vi "EditOptions.vi"(8 "error in":errorcluster, 11 "SequenceNode in":refnum<class "CleanupCategoryNode.lvclass">) -> (0 "error out":errorcluster, 1 "edit options":T1, 2 "subnodes class":T2, 3 "SequenceNode out":refnum<class "CleanupCategoryNode.lvclass">)   [LabVIEW 2015, in "CleanupCategoryNode.lvclass"]
doc: "This VI Contains the options for the Menu that will be displayed when doing right click on an item\nThe subnodes class configures which nodes can be added to this nodes\nAnd the edit options determine which options are available for the node.\n\nThis configuration is stored in this VI in case some dynamic configuration is required for the menu options or subnodes.\n\nAll VIs must overide this methodCopyright 2017 National Instruments Corporation\n\nLicensed under the Apache License, Version 2.0 (the \"License\"); you may not use this file except in compliance with the License. You may obtain a copy of the License at http://www.apache.org/licenses/LICENSE-2.0\nUnless required by applicable law or agreed to in writing, software distributed under the License is distributed on an \"AS IS\" BASIS, WITHOUT WARRANTIES OR CONDITIONS OF ANY KIND, either express or implied. See the License for the specific language governing permissions and limitations under the License."
uses:
  CleanupCategoryNode.lvclass
  <vilib>/NI/Configuration Framework/Node/SubNodeCluster.ctl
  <vilib>/NI/Configuration Framework/Node/NodeMenuOptions.ctl
  <vilib>/NI/Configuration Framework/Node/NISE_CEF_Node.lvclass
  Configuration Tool.lvlib
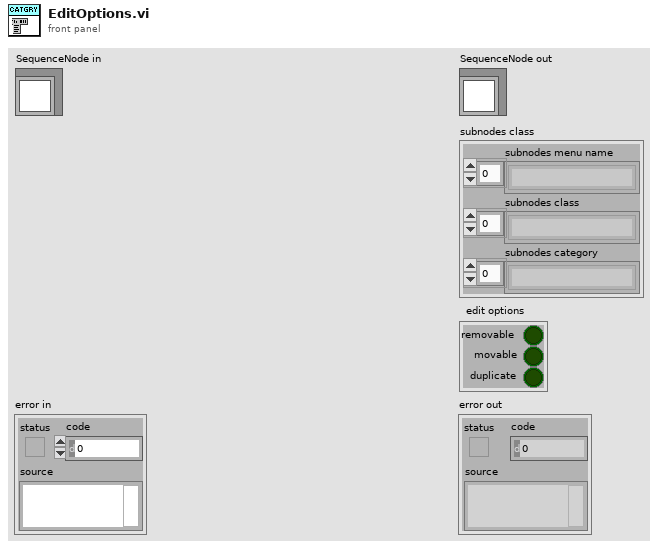
[diagram p1: front panel]
types:
  T1 = typedef "NISE_CEF_Node.lvclass/NodeMenuOptions.ctl" = cluster{"removable":bool, "movable":bool, "duplicate":bool}
  T2 = typedef "NISE_CEF_Node.lvclass/SubNodeCluster.ctl" = cluster{"subnodes menu name":string[], "subnodes class":string[], "subnodes category":string[]}
  T3 = typedef "Configuration Tool.lvlib/StepClassLibrary.ctl" = cluster{"Step Types":string[], "Step Config Classes":refnum<class "Step Config.lvclass">[], "Step UI Classes":refnum<class "Step UI.lvclass">[]}
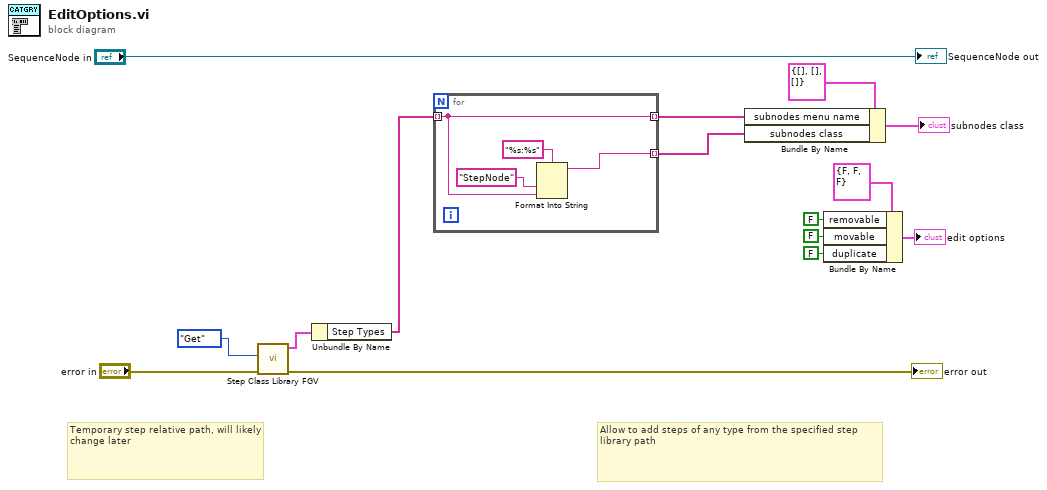
[diagram p0: block diagram]
diagram:
  # "Temporary step relative path, will likely change later"
  # "Allow to add steps of any type from the specified step library path"
  n1 = call "Step Class Library FGV.vi"("error in (no error)"="error in", "Action"=enum16{"Set", "Get"}."Get") -> ("error out"=→"error out":errorcluster, "Step Type Class Library out"=w2:T3)  [unwired: 8 in]
  n2 = Unbundle By Name(w2) -> ("Step Types"=w1:string[])
  n3 = for {
    tunnel: w1 -> [w16] mode=indexing
    tunnel: [w19] -> w6 mode=indexing
    tunnel: [w16] -> w7 mode=indexing
    n4 = Format Into String(format string="%s:%s", "StepNode", w16) -> (resulting string=w19:string)  [unwired: 2 in, 1 out]
  }
  n5 = Bundle By Name(cluster=T2 {"subnodes menu name"=[], "subnodes class"=[], "subnodes category"=[]} ("subnodes class"), "subnodes menu name"=w7, "subnodes class"=w6) -> (→"subnodes class":T2)
  n6 = Bundle By Name(cluster=T1 {"removable"=FALSE, "movable"=FALSE, "duplicate"=FALSE} ("edit options"), "removable"=FALSE ("Removable"), "movable"=FALSE ("Movable"), "duplicate"=FALSE ("Duplicate")) -> (→"edit options":T1)
  "SequenceNode out" <- "SequenceNode in"
